vi "xiC - IMAQ - Exit.vi"(8 "error in (no error)":errorcluster, 11 "Attributes In":T1) -> (0 "error out":errorcluster, 3 "Attributes Out":T1)   [LabVIEW 2015]
uses:
  xiC - IMAQ - Attributes.ctl
  C:/GIT/Cameras3.x/Integrations/Labview/xiLib/xiLIB_32bit/xiLIB/xiCamLib/API/x86/xiApi.NET.dll
  xiLIB_32bit/xiLIB/xiCamLib/API/x86/xiApi.NET.dll
  xiC - IMAQ - TreeDisplayType.ctl
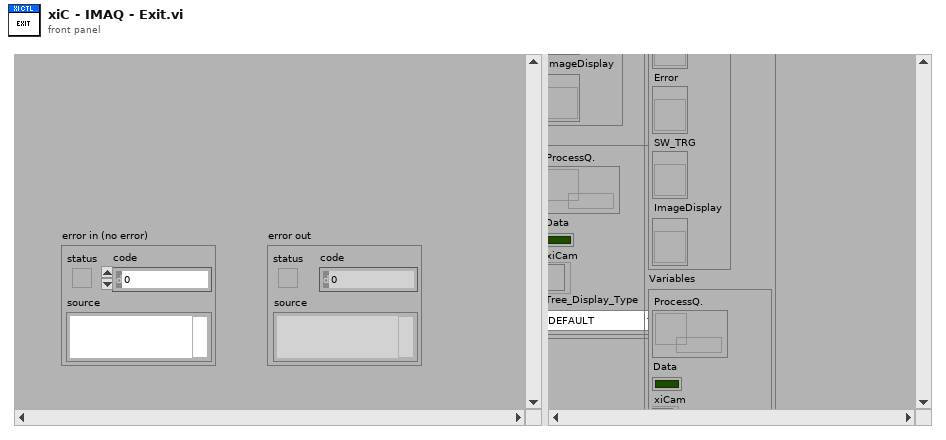
[diagram p1: front panel]
types:
  T1 = typedef "xiC - IMAQ - Attributes.ctl" = cluster{"Controls":cluster{"VI Ref.":refnum<vi>, "Tree":refnum<vi>, "Info":refnum<vi>, "PRMName":refnum<vi>, "xiControl":refnum<vi>, "Error":refnum<vi>, "SW_TRG":refnum<vi>, "ImageDisplay":refnum<vi>}, "Variables":cluster{"ProcessQ.":refnum<queue>, "Data":bool, "xiCam":refnum<k24>, "Tree_Display_Type":T2}}
  T2 = typedef "xiC - IMAQ - TreeDisplayType.ctl" = enum16{"DEFAULT", "HIDE_MAX_MIN"}
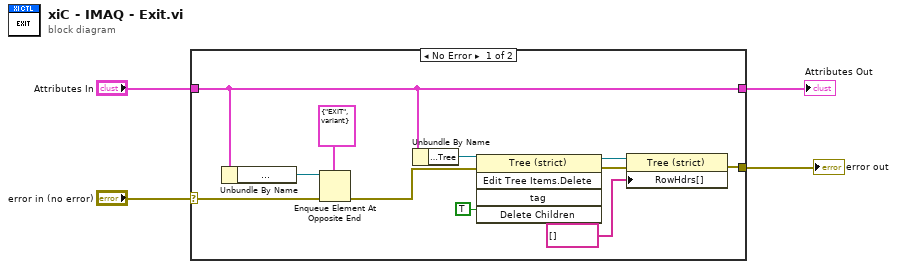
[diagram p0: block diagram]
diagram:
  n1 = case shown="No Error" "error in (no error)" {
    selector: "error in (no error)" -> [w10 w17]
    tunnel: [w6 w17] -> w3
    tunnel: "Attributes In" -> [w13 w16]
    tunnel: [w13 w16] -> w1
    frame No Error {
      n2 = Unbundle By Name(w13) -> ("Variables.ProcessQ."=w12:refnum<queue>)
      n3 = Enqueue Element At Opposite End(queue=w12, element=cluster{"State":string, "Data":variant} {"State"="EXIT", "Data"=variant}, error in (no error)=w10) -> (error out=w11:errorcluster)  [unwired: 1 in, 2 out]
      n4 = Unbundle By Name(w13) -> ("Controls.Tree"=w15:refnum<vi>)
      n5 = invoke class="Tree (strict)" method="Edit Tree Items.Delete"(reference=w15, error in=w11, "Delete Children"=TRUE ("Delete Children?")) -> (reference out=w8:refnum<vi>, error out=w7:errorcluster)  [unwired: 2 in, 3 out]
      n6 = property class="Tree (strict)"(reference=w8, error in=w7, "RowHdrs[]"=string[] [] ("Row Header Strings[]")) -> (error out=w6:errorcluster)  [unwired: 1 out]
    }
    frame Error {
    }
  }
  "error out" <- w3
  "Attributes Out" <- w1
